vi "Test_NotifyStop_StopImmediately_QueuedMessageDropped.vi"(8 "error in (no error)":errorcluster, 11 "TestCase in":refnum<class "TestMessageCycle.lvclass">) -> (0 "error out":errorcluster, 3 "TestCase out":refnum<class "TestMessageCycle.lvclass">)   [LabVIEW 2017, in "TestMessageCycle.lvclass"]
uses:
  TestMessageCycle.lvclass
  Source/MessageCycle/Message Cycle Notifications.ctl
  Source/MessageCycle/MessageCycle.lvclass/MessageCycle.ctl
  <vilib>/ActorFramework/Message Enqueuer/Message Enqueuer.lvclass/Message Enqueuer.ctl
  e7934e2b-a74d-42bd-8965-a9133f77036b.vi
  1b07eade-a78c-42fd-a35c-617bb70b86e5.vi
  <vilib>/ActorFramework/Message Enqueuer/Enqueue.vi
  Doubles/MessageCountsExecutions/MessageCountsExecutions.lvclass
  C:/Program Files (x86)/National Instruments/LabVIEW 2017/vi.lib/ActorFramework/Message/Message.lvclass
  Doubles/ActorCountsMessageCycles/ActorCountsMessageCycles.lvclass
  C:/Program Files (x86)/National Instruments/LabVIEW 2017/vi.lib/ActorFramework/Actor/Actor.lvclass
  Source/MessageCycle/MessageCycle.lvclass
  <vilib>/ActorFramework/Stop Msg/Stop Msg.lvclass
  Source/MessageCycle/Launch Deferred Timeout Notifier.vi
  <vilib>/ActorFramework/Message Priority Queue/Priority Enqueue.vi
  <vilib>/ActorFramework/Message/Message.lvclass
  <vilib>/ActorFramework/Actor/Actor.lvclass
panel:
  out "Cyclic Messages Executed":u32
  out "Cyclic Messages Received":u32
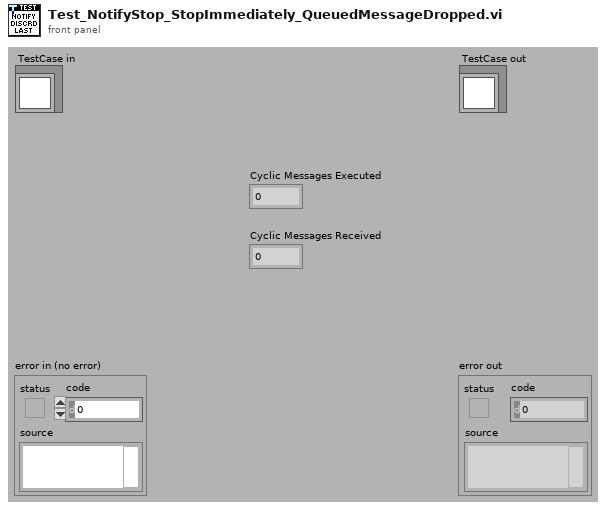
[diagram p1: front panel]
types:
  T1 = typedef "MessageCycle.lvclass/Message Cycle Notifications.ctl" = enum16{"Process Final Copy and Stop", "Stop Immediately", "Substitute Last Message and Stop"}
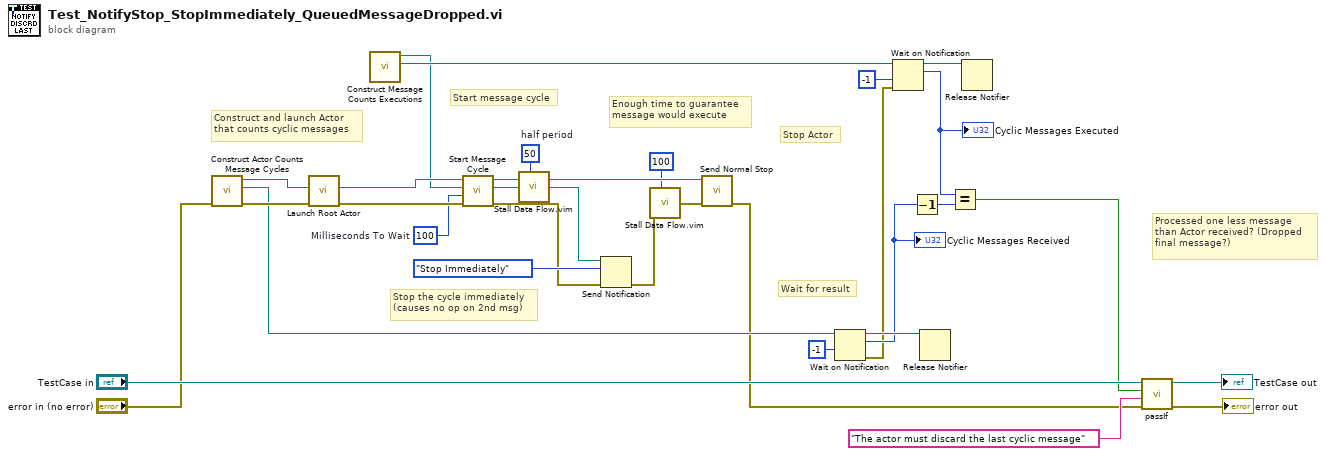
[diagram p0: block diagram]
diagram:
  w12 = u32 50  # half period
  w28 = 100  # Milliseconds To Wait
  # "Enough time to guarantee\nmessage would execute"
  # "Stop the cycle immediately\n(causes no op on 2nd msg)"
  # "Wait for result"
  # "Stop Actor"
  # "Start message cycle"
  # "Processed one less message\nthan Actor received? (Dropped\nfinal message?)"
  # "Construct and launch Actor\nthat counts cyclic messages"
  n1 = call "Construct Actor Counts Message Cycles.vi"("error in (no error)"="error in (no error)") -> ("error out"=w21:errorcluster, "Final Count"=w20:refnum<notifier>, "ActorCountsMessageCycles"=w23:refnum<class "ActorCountsMessageCycles.lvclass">)  [unwired: 8 in]
  n2 = call <vilib>:"Launch Root Actor.vi"("error in (no error)"=w21, "Actor"=w23) -> ("error out"=w32:errorcluster, "Actor's Enqueuer"=w27:refnum<class "Message Enqueuer.lvclass">)  [unwired: 8 in]
  n3 = call "Construct Message Counts Executions.vi"() -> ("Message Executions"=w5:refnum<notifier>, "CyclicMessageCountsCycles out"=w1:refnum<class "MessageCountsExecutions.lvclass">)  [unwired: 9 in, 1 out]
  n4 = call "Start Message Cycle.vi"("error in (no error)"=w32, "Inter-Message Wait [ms] (0)"=w28, "Message"=w1, "Message Enqueuer"=w27) -> ("error out"=w11:errorcluster, "Message Cycle Notifier"=w15:refnum<notifier>, "Message Enqueuer out"=w26:refnum<class "Message Enqueuer.lvclass">)  [unwired: 5 in]
  n5 = call "Stall Data Flow.vim"("value in"=w15, "milliseconds to wait"=w12) -> ("value out"=w13:refnum<notifier>)  [unwired: 1 out]
  n6 = Send Notification(notification=Message_Cycle_Notifications."Stop Immediately", notifier=w13, error in (no error)=w11) -> (error out=w10:errorcluster)  [unwired: 1 out]
  n7 = call "Stall Data Flow.vim"("value in"=w10, "milliseconds to wait"=u32 100) -> ("value out"=w9:errorcluster)  [unwired: 1 out]
  n8 = call <vilib>:"Send Normal Stop.vi"("error in (no error)"=w9, "Message Enqueuer"=w26) -> ("error out"=w17:errorcluster)  [unwired: 9 in]
  n9 = Wait on Notification(notifier=w20, timeout in ms (-1)=-1) -> (notifier out=w18:refnum<notifier>, notification=w16:u32, error out=w6:errorcluster)  [unwired: 2 in, 1 out]
  "Cyclic Messages Received" <- w16
  n10 = Wait on Notification(notifier=w5, timeout in ms (-1)=-1, error in (no error)=w6) -> (notifier out=w4:refnum<notifier>, notification=w3:u32)  [unwired: 1 in, 2 out]
  "Cyclic Messages Executed" <- w3
  n11 = Decrement(x=w16) -> (x-1=w2:u32)
  n12 = Release Notifier(notifier=w18) -> ()  [unwired: 2 in, 3 out]
  n13 = Equal?(x=w3, y=w2) -> (x = y?=w25:bool)
  n14 = Release Notifier(notifier=w4) -> ()  [unwired: 2 in, 3 out]
  n15 = call-dynamic "passIf.vi"("error in (no error)"=w17, "message (\"\")"="The actor must discard the last cyclic message" ("message (\"\")"), "pass"=w25, "TestCase in"="TestCase in") -> ("error out"=→"error out":errorcluster, "TestCase out"=→"TestCase out":refnum<class "TestMessageCycle.lvclass">)  [unwired: 6 in]
